vi "rszvl_core_global.vi"() -> ()   [LabVIEW 2014] (continued)
Callback"="", "Range Callback"="", "Check Callback"="", "Rngtable Callback"="", "Coerce Callback"="", "User Callback"="", "Supported Models"="", "Instrument Options"="", "Repeated Capabilities"="", "Restricted Repeated Capabilities"="", "Help"="This attribute sets the level when AM–modulated signals are used as trigger source.\n\nAvailable Repeated Capabilities:\nNone\n\nRemote-control command(s):\nTRIGger<1|2>[:SEQuence]:LEVel:AM:RELative", "Flags"={"OPC Wait"=FALSE, "Dont check status"=FALSE, "*WAI"=FALSE}, "Check Status Callback"=""}, {"Level"=2, "Descriptive Name"="Analog Demod Trigger FM Level", "Class Only"=FALSE, "Data Type"=1, "Access"=2, "Identifier"="RSZVL_ATTR_ADEM_TRIGGER_FM_LEVEL", "Range Table"="rszvl_rngAdemTrigFMLevel", "Command"="TRIG:LEV:FM", "Read Callback"="", "Write Callback"="", "Range Callback"="", "Check Callback"="", "Rngtable Callback"="", "Coerce Callback"="", "User Callback"="", "Supported Models"="", "Instrument Options"="", "Repeated Capabilities"="", "Restricted Repeated Capabilities"="", "Help"="This attribute sets the level when FM–modulated signals are used as trigger source.\n\nAvailable Repeated Capabilities:\nNone\n\nRemote-control command(s):\nTRIGger<1|2>[:SEQuence]:LEVel:FM", "Flags"={"OPC Wait"=FALSE, "Dont check status"=FALSE, "*WAI"=FALSE}, "Check Status Callback"=""}, {"Level"=2, "Descriptive Name"="Analog Demod Trigger PM Level", "Class Only"=FALSE, "Data Type"=1, "Access"=2, "Identifier"="RSZVL_ATTR_ADEM_TRIGGER_PM_LEVEL", "Range Table"="rszvl_rngAdemTrigPMLevel", "Command"="TRIG:LEV:PM", "Read Callback"="", "Write Callback"="", "Range Callback"="", "Check Callback"="", "Rngtable Callback"="", "Coerce Callback"="", "User Callback"="", "Supported Models"="", "Instrument Options"="", "Repeated Capabilities"="", "Restricted Repeated Capabilities"="", "Help"="This attribute sets the level when PM–modulated signals are used as trigger source.\n\nAvailable Repeated Capabilities:\nNone\n\nRemote-control command(s):\nTRIGger<1|2>[:SEQuence]:LEVel:PM", "Flags"={"OPC Wait"=FALSE, "Dont check status"=FALSE, "*WAI"=FALSE}, "Check Status Callback"=""}, {"Level"=2, "Descriptive Name"="Settings", "Class Only"=TRUE, "Data Type"=0, "Access"=0, "Identifier"="", "Range Table"="", "Command"="", "Read Callback"="", "Write Callback"="", "Range Callback"="", "Check Callback"="", "Rngtable Callback"="", "Coerce Callback"="", "User Callback"="", "Supported Models"="", "Instrument Options"="", "Repeated Capabilities"="", "Restricted Repeated Capabilities"="", "Help"="Attributes that configures the common settings of FM Demodulator.\n\n(1) FM Demod Display Pdiv:\nThis attribute defines the scaling of the Y axis in the current unit.\n\n(2) FM Demod State:\nThis attribute activates the FM demodulator of the instrument. The instrument will be set to timedomain\nmeasurement (span = 0) at the current center frequency. The detector will be set to\nSAMPle, the demodulator itself will be set up according to the parameters of command\n[SENSe:]ADEMod:SET.\n\n(3) FM Demod AF Coupling:\nThis attribute selects the coupling of the AF path.\n\n(4) FM Demod Meas Time:\nThis attribute sets the measuring time for the analog demodulation.\n\n(5) FM Demod Bandwidth:\nThis attribute defines the demodulation bandwidth for analog demodulation. Depending on the selected demodulation bandwidth, the instrument selects the required sampling rate.\nThe available values of the demodulation bandwidths are defined by the sampling rates.\n\n(6) FM Demod Record Length:\nThis attribute returns the currently set record length for the analog demodulation.\n\n(7) FM Demod Sampling Rate:\nThis attribute returns the currently set sampling rate for the analog demodulation.\n\n(8) FM Demod Zoom State:\nThis attribute switches on or off the zoom function for the trace data of the FM demodulator.\nDepending on the selected measuring time and demodulation bandwidth, more test points are recorded than can be displayed.\n\n(9) FM Demod Zoom Start:\nThis attribute selects the start time for the display of the single measured values of the FM\ndemodulator.\n\n(10) Analog Demod Phase Wrap:\nThis attribute activates the limitation to ±180°.\n\n(11) Analog Demod Unit Angle:\nThis attribute selects the unit for angles.\n\n(12) Analog Demod Zero Phase Ref Point:\nThis attribute activates the input of the reference point, where the phase is set to 0 rad.\n\n(13) Analog Demod THD Unit:\nThis attribute selects the unit for THD measurement results.", "Flags"={"OPC Wait"=FALSE, "Dont check status"=FALSE, "*WAI"=FALSE}, "Check Status Callback"=""}, {"Level"=3, "Descriptive Name"="FM Demod Display Pdiv", "Class Only"=FALSE, "Data Type"=1, "Access"=2, "Identifier"="RSZVL_ATTR_FMDEM_DISPLAY_PDIV", "Range Table"="", "Command"="DISP:WIND:TRAC:Y:PDIV", "Read Callback"="", "Write Callback"="", "Range Callback"="", "Check Callback"="", "Rngtable Callback"="", "Coerce Callback"="", "User Callback"="", "Supported Models"="", "Instrument Options"="", "Repeated Capabilities"="", "Restricted Repeated Capabilities"="", "Help"="This attribute defines the scaling of the Y axis in the current unit.\n\nAvailable Repeated Capabilities:\nNone\n\nRemote-control command(s):\nDISPlay[:WINDow<1|2>]:TRACE<1 to 3>:Y[:SCALe]:PDIVision", "Flags"={"OPC Wait"=FALSE, "Dont check status"=FALSE, "*WAI"=FALSE}, "Check Status Callback"=""}, {"Level"=3, "Descriptive Name"="FM Demod State", "Class Only"=FALSE, "Data Type"=3, "Access"=2, "Identifier"="RSZVL_ATTR_FMDEM_STATE", "Range Table"="", "Command"="ADEM", "Read Callback"="", "Write Callback"="", "Range Callback"="", "Check Callback"="", "Rngtable Callback"="", "Coerce Callback"="", "User Callback"="", "Supported Models"="", "Instrument Options"="", "Repeated Capabilities"="", "Restricted Repeated Capabilities"="", "Help"="This attribute activates the FM demodulator of the instrument. The instrument will be set to timedomain\nmeasurement (span = 0) at the current center frequency. The detector will be set to\nSAMPle, the demodulator itself will be set up according to the parameters of command\n[SENSe:]ADEMod:SET.\n\nAvailable Repeated Capabilities:\nNone\n\nRemote-control command(s):\n[SENSe:]ADEMod[:STATe] ON | OFF", "Flags"={"OPC Wait"=FALSE, "Dont check status"=FALSE, "*WAI"=FALSE}, "Check Status Callback"=""}, {"Level"=3, "Descriptive Name"="FM Demod AF Coupling", "Class Only"=FALSE, "Data Type"=0, "Access"=2, "Identifier"="RSZVL_ATTR_FMDEM_AF_COUP", "Range Table"="rszvl_rngCoupling", "Command"="ADEM:AF:COUP", "Read Callback"="", "Write Callback"="", "Range Callback"="", "Check Callback"="", "Rngtable Callback"="", "Coerce Callback"="", "User Callback"="", "Supported Models"="", "Instrument Options"="", "Repeated Capabilities"="", "Restricted Repeated Capabilities"="", "Help"="This attribute selects the coupling of the AF path.\n\nAvailable Repeated Capabilities:\nNone\n\nRemote-control command(s):\n[SENSe:]ADEMod:AF:COUPling AC | DC", "Flags"={"OPC Wait"=FALSE, "Dont check status"=FALSE, "*WAI"=FALSE}, "Check Status Callback"=""}, {"Level"=3, "Descriptive Name"="FM Demod Meas Time", "Class Only"=FALSE, "Data Type"=1, "Access"=2, "Identifier"="RSZVL_ATTR_FMDEM_MTIM", "Range Table"="", "Command"="ADEM:MTIM", "Read Callback"="", "Write Callback"="", "Range Callback"="", "Check Callback"="", "Rngtable Callback"="", "Coerce Callback"="", "User Callback"="", "Supported Models"="", "Instrument Options"="", "Repeated Capabilities"="", "Restricted Repeated Capabilities"="", "Help"="This attribute sets the measuring time for the analog demodulation.\n\nAvailable Repeated Capabilities:\nNone\n\nRemote-control command(s):\n[SENSe:]ADEMod:MTIMe", "Flags"={"OPC Wait"=FALSE, "Dont check status"=FALSE, "*WAI"=FALSE}, "Check Status Callback"=""}, {"Level"=3, "Descriptive Name"="FM Demod Bandwidth", "Class Only"=FALSE, "Data Type"=1, "Access"=2, "Identifier"="RSZVL_ATTR_FMDEM_BAND_DEM", "Range Table"="rszvl_rngFmBwid", "Command"="ADEM:BAND:DEM", "Read Callback"="", "Write Callback"="", "Range Callback"="", "Check Callback"="", "Rngtable Callback"="", "Coerce Callback"="", "User Callback"="", "Supported Models"="", "Instrument Options"="", "Repeated Capabilities"="", "Restricted Repeated Capabilities"="", "Help"="This attribute defines the demodulation bandwidth for analog demodulation. Depending on the selected demodulation bandwidth, the instrument selects the required sampling rate.\nThe available values of the demodulation bandwidths are defined by the sampling rates.\n\nAvailable Repeated Capabilities:\nNone\n\nRemote-control command(s):\n[SENSe:]ADEMod:BANDwidth | BWIDth:DEModulation", "Flags"={"OPC Wait"=FALSE, "Dont check status"=FALSE, "*WAI"=FALSE}, "Check Status Callback"=""}, {"Level"=3, "Descriptive Name"="FM Demod Record Length", "Class Only"=FALSE, "Data Type"=1, "Access"=0, "Identifier"="RSZVL_ATTR_FMDEM_RLEN", "Range Table"="", "Command"="ADEM:RLEN?", "Read Callback"="", "Write Callback"="", "Range Callback"="", "Check Callback"="", "Rngtable Callback"="", "Coerce Callback"="", "User Callback"="", "Supported Models"="", "Instrument Options"="", "Repeated Capabilities"="", "Restricted Repeated Capabilities"="", "Help"="This attribute returns the currently set record length for the analog demodulation.\n\nAvailable Repeated Capabilities:\nNone\n\nRemote-control command(s):\n[SENSe:]ADEMod:RLENgth?", "Flags"={"OPC Wait"=FALSE, "Dont check status"=FALSE, "*WAI"=FALSE}, "Check Status Callback"=""}, {"Level"=3, "Descriptive Name"="FM Demod Sampling Rate", "Class Only"=FALSE, "Data Type"=1, "Access"=0, "Identifier"="RSZVL_ATTR_FMDEM_SRATE", "Range Table"="", "Command"="ADEM:SRAT?", "Read Callback"="", "Write Callback"="", "Range Callback"="", "Check Callback"="", "Rngtable Callback"="", "Coerce Callback"="", "User Callback"="", "Supported Models"="", "Instrument Options"="", "Repeated Capabilities"="", "Restricted Repeated Capabilities"="", "Help"="This attribute returns the currently set sampling rate for the analog demodulation.\n\nAvailable Repeated Capabilities:\nNone\n\nRemote-control command(s):\n[SENSe:]ADEMod:SRATe?", "Flags"={"OPC Wait"=FALSE, "Dont check status"=FALSE, "*WAI"=FALSE}, "Check Status Callback"=""}, {"Level"=3, "Descriptive Name"="FM Demod Zoom State", "Class Only"=FALSE, "Data Type"=3, "Access"=2, "Identifier"="RSZVL_ATTR_FMDEM_ZOOM", "Range Table"="", "Command"="ADEM:ZOOM", "Read Callback"="", "Write Callback"="", "Range Callback"="", "Check Callback"="", "Rngtable Callback"="", "Coerce Callback"="", "User Callback"="", "Supported Models"="", "Instrument Options"="", "Repeated Capabilities"="", "Restricted Repeated Capabilities"="", "Help"="This attribute switches on or off the zoom function for the trace data of the FM demodulator.\nDepending on the selected measuring time and demodulation bandwidth, more test points are recorded than can be displayed.\n\nAvailable Repeated Capabilities:\nNone\n\nRemote-control command(s):\n[SENSe:]ADEMod:ZOOM[:STATe] ON | OFF", "Flags"={"OPC Wait"=FALSE, "Dont check status"=FALSE, "*WAI"=FALSE}, "Check Status Callback"=""}, {"Level"=3, "Descriptive Name"="FM Demod Zoom Start", "Class Only"=FALSE, "Data Type"=1, "Access"=2, "Identifier"="RSZVL_ATTR_FMDEM_ZOOM_START", "Range Table"="", "Command"="ADEM:ZOOM:STAR", "Read Callback"="", "Write Callback"="", "Range Callback"="", "Check Callback"="", "Rngtable Callback"="", "Coerce Callback"="", "User Callback"="", "Supported Models"="", "Instrument Options"="", "Repeated Capabilities"="", "Restricted Repeated Capabilities"="", "Help"="This attribute selects the start time for the display of the single measured values of the FM\ndemodulator.\n\nAvailable Repeated Capabilities:\nNone\n\nRemote-control command(s):\n[SENSe:]ADEMod:ZOOM:STARt", "Flags"={"OPC Wait"=FALSE, "Dont check status"=FALSE, "*WAI"=FALSE}, "Check Status Callback"=""}, {"Level"=3, "Descriptive Name"="Analog Demod Phase Wrap", "Class Only"=FALSE, "Data Type"=0, "Access"=2, "Identifier"="RSZVL_ATTR_ADEM_PHASE_WRAP", "Range Table"="rszvl_rngAdemPhaseWrap", "Command"="CALC:FORM", "Read Callback"="", "Write Callback"="", "Range Callback"="", "Check Callback"="", "Rngtable Callback"="", "Coerce Callback"="", "User Callback"="", "Supported Models"="", "Instrument Options"="", "Repeated Capabilities"="", "Restricted Repeated Capabilities"="", "Help"="This attribute activates the limitation to ±180°.\n\nAvailable Repeated Capabilities:\nNone\n\nRemote-control command(s):\nCALCulate<1|2>:FORMat", "Flags"={"OPC Wait"=FALSE, "Dont check status"=FALSE, "*WAI"=FALSE}, "Check Status Callback"=""}, {"Level"=3, "Descriptive Name"="Analog Demod Unit Angle", "Class Only"=FALSE, "Data Type"=0, "Access"=2, "Identifier"="RSZVL_ATTR_ADEM_UNIT_ANGLE", "Range Table"="rszvl_rngUnitAngle", "Command"="CALC:UNIT:ANGL", "Read Callback"="", "Write Callback"="", "Range Callback"="", "Check Callback"="", "Rngtable Callback"="", "Coerce Callback"="", "User Callback"="", "Supported Models"="", "Instrument Options"="", "Repeated Capabilities"="", "Restricted Repeated Capabilities"="", "Help"="This attribute selects the unit for angles.\n\nAvailable Repeated Capabilities:\nNone\n\nRemote-control command(s):\nCALCulate<1|2>:UNIT:ANGLe", "Flags"={"OPC Wait"=FALSE, "Dont check status"=FALSE, "*WAI"=FALSE}, "Check Status Callback"=""}, {"Level"=3, "Descriptive Name"="Analog Demod Zero Phase Ref Point", "Class Only"=FALSE, "Data Type"=1, "Access"=2, "Identifier"="RSZVL_ATTR_ADEM_PM_RPO_X", "Range Table"="", "Command"="ADEM:PM:RPO:X", "Read Callback"="", "Write Callback"="", "Range Callback"="", "Check Callback"="", "Rngtable Callback"="", "Coerce Callback"="", "User Callback"="", "Supported Models"="", "Instrument Options"="", "Repeated Capabilities"="", "Restricted Repeated Capabilities"="", "Help"="This attribute activates the input of the reference point, where the phase is set to 0 rad.\n\nAvailable Repeated Capabilities:\nNone\n\nRemote-control command(s):\n[SENSe1:]ADEMod:PM:RPO:X", "Flags"={"OPC Wait"=FALSE, "Dont check status"=FALSE, "*WAI"=FALSE}, "Check Status Callback"=""}, {"Level"=2, "Descriptive Name"="AF Frequency Settings", "Class Only"=TRUE, "Data Type"=0, "Access"=0, "Identifier"="", "Range Table"="", "Command"="", "Read Callback"="", "Write Callback"="", "Range Callback"="", "Check Callback"="", "Rngtable Callback"="", "Coerce Callback"="", "User Callback"="", "Supported Models"="", "Instrument Options"="", "Repeated Capabilities"="", "Restricted Repeated Capabilities"="", "Help"="Attributes that configures the AF Frequency settings.\n\n(1) FM Demod AF Center Frequency:\nThis attribute sets the center frequency for result display AF spectrum.\n\n(2) FM Demod AF Span:\nThis attribute sets the span for result display AF spectrum.\nThe span is limited to half the measurement bandwidth of analog demodulation.\n\n(3) FM Demod AF Start Frequency:\nThis attribute sets the start frequency for result display AF spectrum.\n\n(4) FM Demod AF Stop Frequency:\nThis attribute sets the stop frequency for result display AF spectrum.\nThe stop frequency is limited to half the measurement bandwidth of analog demodulation.\n\n(5) FM Demod AF Full Span:\nThis attribute sets the maximum span for the display of the AF spectrum.", "Flags"={"OPC Wait"=FALSE, "Dont check status"=FALSE, "*WAI"=FALSE}, "Check Status Callback"=""}, {"Level"=3, "Descriptive Name"="FM Demod AF Center Frequency", "Class Only"=FALSE, "Data Type"=1, "Access"=2, "Identifier"="RSZVL_ATTR_FMDEM_AF_CENTER", "Range Table"="", "Command"="ADEM:AF:CENT", "Read Callback"="", "Write Callback"="", "Range Callback"="", "Check Callback"="", "Rngtable Callback"="", "Coerce Callback"="", "User Callback"="", "Supported Models"="", "Instrument Options"="", "Repeated Capabilities"="", "Restricted Repeated Capabilities"="", "Help"="This attribute sets the center frequency for result display AF spectrum.\n\nAvailable Repeated Capabilities:\nNone\n\nRemote-control command(s):\n[SENSe:]ADEMod:AF:CENTer", "Flags"={"OPC Wait"=FALSE, "Dont check status"=FALSE, "*WAI"=FALSE}, "Check Status Callback"=""}, {"Level"=3, "Descriptive Name"="FM Demod AF Span", "Class Only"=FALSE, "Data Type"=1, "Access"=2, "Identifier"="RSZVL_ATTR_FMDEM_AF_SPAN", "Range Table"="", "Command"="ADEM:AF:SPAN", "Read Callback"="", "Write Callback"="", "Range Callback"="", "Check Callback"="", "Rngtable Callback"="", "Coerce Callback"="", "User Callback"="", "Supported Models"="", "Instrument Options"="", "Repeated Capabilities"="", "Restricted Repeated Capabilities"="", "Help"="This attribute sets the span for result display AF spectrum.\nThe span is limited to half the measurement bandwidth of analog demodulation.\n\nAvailable Repeated Capabilities:\nNone\n\nRemote-control command(s):\n[SENSe:]ADEMod:AF:SPAN", "Flags"={"OPC Wait"=FALSE, "Dont check status"=FALSE, "*WAI"=FALSE}, "Check Status Callback"=""}, {"Level"=3, "Descriptive Name"="FM Demod AF Start Frequency", "Class Only"=FALSE, "Data Type"=1, "Access"=2, "Identifier"="RSZVL_ATTR_FMDEM_AF_START", "Range Table"="", "Command"="ADEM:AF:STAR", "Read Callback"="", "Write Callback"="", "Range Callback"="", "Check Callback"="", "Rngtable Callback"="", "Coerce Callback"="", "User Callback"="", "Supported Models"="", "Instrument Options"="", "Repeated Capabilities"="", "Restricted Repeated Capabilities"="", "Help"="This attribute sets the start frequency for result display AF spectrum.\n\nAvailable Repeated Capabilities:\nNone\n\nRemote-control command(s):\n[SENSe:]ADEMod:AF:STARt", "Flags"={"OPC Wait"=FALSE, "Dont check status"=FALSE, "*WAI"=FALSE}, "Check Status Callback"=""}, {"Level"=3, "Descriptive Name"="FM Demod AF Stop Frequency", "Class Only"=FALSE, "Data Type"=1, "Access"=2, "Identifier"="RSZVL_ATTR_FMDEM_AF_STOP", "Range Table"="", "Command"="ADEM:AF:STOP", "Read Callback"="", "Write Callback"="", "Range Callback"="", "Check Callback"="", "Rngtable Callback"="", "Coerce Callback"="", "User Callback"="", "Supported Models"="", "Instrument Options"="", "Repeated Capabilities"="", "Restricted Repeated Capabilities"="", "Help"="This attribute sets the stop frequency for result display AF spectrum.\nThe stop frequency is limited to half the measurement bandwidth of analog demodulation.\n\nAvailable Repeated Capabilities:\nNone\n\nRemote-control command(s):\n[SENSe:]ADEMod:AF:STOP", "Flags"={"OPC Wait"=FALSE, "Dont check status"=FALSE, "*WAI"=FALSE}, "Check Status Callback"=""}, {"Level"=3, "Descriptive Name"="FM Demod AF Full Span", "Class Only"=FALSE, "Data Type"=4, "Access"=1, "Identifier"="RSZVL_ATTR_FMDEM_AF_FULL_SPAN", "Range Table"="", "Command"="ADEM:AF:SPAN:FULL", "Read Callback"="", "Write Callback"="", "Range Callback"="", "Check Callback"="", "Rngtable Callback"="", "Coerce Callback"="", "User Callback"="", "Supported Models"="", "Instrument Options"="", "Repeated Capabilities"="", "Restricted Repeated Capabilities"="", "Help"="This attribute sets the maximum span for the display of the AF spectrum.\n\nAvailable Repeated Capabilities:\nNone\n\nRemote-control command(s):\n[SENSe:]ADEMod:AF:SPAN:FULL", "Flags"={"OPC Wait"=FALSE, "Dont check status"=FALSE, "*WAI"=FALSE}, "Check Status Callback"=""}, {"Level"=2, "Descriptive Name"="RF Spectrum Settings", "Class Only"=TRUE, "Data Type"=0, "Access"=0, "Identifier"="", "Range Table"="", "Command"="", "Read Callback"="", "Write Callback"="", "Range Callback"="", "Check Callback"="", "Rngtable Callback"="", "Coerce Callback"="", "User Callback"="", "Supported Models"="", "Instrument Options"="", "Repeated Capabilities"="", "Restricted Repeated Capabilities"="", "Help"="Attributes that configures the RF Spectrum settings.\n\n(1) FM Demod RF Spectrum Resolution Bandwidth:\nThis attribute sets the resolution bandwidth for display of the RF spectrum from the data of analog\ndemodulation.\nThe required record length is calculated from the sampling rate directly set via\nADEM:SPEC:SPAN:MAX or ADEM:BAND. If the available record length is not sufficient for the\ngiven bandwidth, it is set to maximum and the resolution bandwidth is increased accordingly.\n\n(2) FM Demod RF Spectrum Span:\nThis attribute sets the maximum frequency range for result display of RF spectrum resulting from\nthe FM demodulation data. The maximum span corresponds to the measurement bandwidth of\nanalog demodulation (SENS:ADEM:BAND).\n\n(3) FM Demod RF Spectrum Zoom:\nThis attribute sets the frequency range for result display of RF spectrum determined from FM demodulation data. The frequency range for result display is limited to the maximum span or to the measurement  bandwidth of analog demodulation.", "Flags"={"OPC Wait"=FALSE, "Dont check status"=FALSE, "*WAI"=FALSE}, "Check Status Callback"=""}, {"Level"=3, "Descriptive Name"="FM Demod RF Spectrum Resolution Bandwidth", "Class Only"=FALSE, "Data Type"=1, "Access"=2, "Identifier"="RSZVL_ATTR_FMDEM_BAND_RES", "Range Table"="rszvl_rngAdemBandRes", "Command"="ADEM:SPEC:BAND", "Read Callback"="", "Write Callback"="", "Range Callback"="", "Check Callback"="", "Rngtable Callback"="", "Coerce Callback"="", "User Callback"="", "Supported Models"="", "Instrument Options"="", "Repeated Capabilities"="", "Restricted Repeated Capabilities"="", "Help"="This attribute sets the resolution bandwidth for display of the RF spectrum from the data of analog\ndemodulation.\nThe required record length is calculated from the sampling rate directly set via\nADEM:SPEC:SPAN:MAX or ADEM:BAND. If the available record length is not sufficient for the\ngiven bandwidth, it is set to maximum and the resolution bandwidth is increased accordingly.\n\nAvailable Repeated Capabilities:\nNone\n\nRemote-control command(s):\n[SENSe:]ADEMod:SPECtrum:BANDwidth|BWIDth[:RESolution]", "Flags"={"OPC Wait"=FALSE, "Dont check status"=FALSE, "*WAI"=FALSE}, "Check Status Callback"=""}, {"Level"=3, "Descriptive Name"="FM Demod RF Spectrum Span", "Class Only"=FALSE, "Data Type"=1, "Access"=2, "Identifier"="RSZVL_ATTR_FMDEM_SPEC_SPAN", "Range Table"="", "Command"="ADEM:SPEC:SPAN", "Read Callback"="", "Write Callback"="", "Range Callback"="", "Check Callback"="", "Rngtable Callback"="", "Coerce Callback"="", "User Callback"="", "Supported Models"="", "Instrument Options"="", "Repeated Capabilities"="", "Restricted Repeated Capabilities"="", "Help"="This attribute sets the maximum frequency range for result display of RF spectrum resulting from\nthe FM demodulation data. The maximum span corresponds to the measurement bandwidth of\nanalog demodulation (SENS:ADEM:BAND).\n\nAvailable Repeated Capabilities:\nNone\n\nRemote-control command(s):\n[SENSe:]ADEMod:SPECtrum:SPAN[:MAXimum]", "Flags"={"OPC Wait"=FALSE, "Dont check status"=FALSE, "*WAI"=FALSE}, "Check Status Callback"=""}, {"Level"=3, "Descriptive Name"="FM Demod RF Spectrum Zoom", "Class Only"=FALSE, "Data Type"=1, "Access"=2, "Identifier"="RSZVL_ATTR_FMDEM_SPEC_ZOOM", "Range Table"="", "Command"="ADEM:SPEC:SPAN:ZOOM", "Read Callback"="", "Write Callback"="", "Range Callback"="", "Check Callback"="", "Rngtable Callback"="", "Coerce Callback"="", "User Callback"="", "Supported Models"="", "Instrument Options"="", "Repeated Capabilities"="", "Restricted Repeated Capabilities"="", "Help"="This attribute sets the frequency range for result display of RF spectrum determined from FM demodulation data. The frequency range for result display is limited to the maximum span or to the measurement  bandwidth of analog demodulation.\n\nAvailable Repeated Capabilities:\nNone\n\nRemote-control command(s):\n[SENSe:]ADEMod:SPECtrum:SPAN:ZOOM", "Flags"={"OPC Wait"=FALSE, "Dont check status"=FALSE, "*WAI"=FALSE}, "Check Status Callback"=""}, {"Level"=2, "Descriptive Name"="AF Filter Settings", "Class Only"=TRUE, "Data Type"=0, "Access"=0, "Identifier"="", "Range Table"="", "Command"="", "Read Callback"="", "Write Callback"="", "Range Callback"="", "Check Callback"="", "Rngtable Callback"="", "Coerce Callback"="", "User Callback"="", "Supported Models"="", "Instrument Options"="", "Repeated Capabilities"="", "Restricted Repeated Capabilities"="", "Help"="Attributes that configures the AF Filter settings.\n\n(1) FM Demod High Pass AF Filter State:\nThis attribute switches on a high pass filter with the given limit to separate the DC component.\n\n(2) FM Demod High Pass AF Filter Frequency:\nThis attribute sets the limit of high pass filter to separate the DC component. The filters are indicated by the 3 dB cutoff frequency. The filters are designed as 2nd-order Butterworth filter (12 dB/octave).\n\n(3) FM Demod Low Pass AF Filter State:\nThis attribute switches on/off a low pass filter.\n\n(4) FM Demod Deemphasis State:\nThis attribute switches on/off the de-emphasis.\n\n(5) FM Demod Low Pass AF Filter Frequency:\nThis attribute sets the limit of low pass filter. The filter are indicated by the 3 dB cutoff frequency. The 3 kHz and 15 kHz filters are designed as 5th-order Butterworth filter (30 dB/octave). The\n150 kHz filter is designed as 8th-order Butterworth filter (48 dB/octave).\n\n(6) FM Demod Deemphasis Time Constant:\nThis attribute sets the de-emphasisi time constant.\n\n(7) Analog Demod Low Pass Filter Frequency Relative:\nThis attribute selects the relative low pass filter type.\n\n(8) Analog Demod Filter CCITT Weighting:\nThis attribute activates/deactivate CCITT filter weightening. \nCCITT 25 kHz <= demodulation bandwidth <= 3 MHz\n\n(9) Analog Demod Filter CCIR Weighting:\nThis attribute activates/deactivate CCIR filter weightening. \nCCIR 50 kHz <= demodulation bandwidth <= 1.6 MHz", "Flags"={"OPC Wait"=FALSE, "Dont check status"=FALSE, "*WAI"=FALSE}, "Check Status Callback"=""}, {"Level"=3, "Descriptive Name"="FM Demod High Pass AF Filter State", "Class Only"=FALSE, "Data Type"=3, "Access"=2, "Identifier"="RSZVL_ATTR_FMDEM_FILT_HPAS_STAT", "Range Table"="", "Command"="FILT:HPAS", "Read Callback"="", "Write Callback"="", "Range Callback"="", "Check Callback"="", "Rngtable Callback"="", "Coerce Callback"="", "User Callback"="", "Supported Models"="", "Instrument Options"="", "Repeated Capabilities"="", "Restricted Repeated Capabilities"="", "Help"="This attribute switches on a high pass filter with the given limit to separate the DC component.\n\nAvailable Repeated Capabilities:\nNone\n\nRemote-control command(s):\n[SENSe:]FILTer:HPASs[:STATe] ON | OFF", "Flags"={"OPC Wait"=FALSE, "Dont check status"=FALSE, "*WAI"=FALSE}, "Check Status Callback"=""}, {"Level"=3, "Descriptive Name"="FM Demod High Pass AF Filter Frequency", "Class Only"=FALSE, "Data Type"=1, "Access"=2, "Identifier"="RSZVL_ATTR_FMDEM_FILT_HPAS_FREQ", "Range Table"="rszvl_rngHpasFilterFreq", "Command"="FILT:HPAS:FREQ", "Read Callback"="", "Write Callback"="", "Range Callback"="", "Check Callback"="", "Rngtable Callback"="", "Coerce Callback"="", "User Callback"="", "Supported Models"="", "Instrument Options"="", "Repeated Capabilities"="", "Restricted Repeated Capabilities"="", "Help"="This attribute sets the limit of high pass filter to separate the DC component. The filters are indicated by the 3 dB cutoff frequency. The filters are designed as 2nd-order Butterworth filter (12 dB/octave).\n\nAvailable Repeated Capabilities:\nNone\n\nRemote-control command(s):\n[SENSe:]FILTer:HPASs:FREQuency 50 Hz | 300 Hz", "Flags"={"OPC Wait"=FALSE, "Dont check status"=FALSE, "*WAI"=FALSE}, "Check Status Callback"=""}, {"Level"=3, "Descriptive Name"="FM Demod Low Pass AF Filter State", "Class Only"=FALSE, "Data Type"=3, "Access"=2, "Identifier"="RSZVL_ATTR_FMDEM_FILT_LPAS_STAT", "Range Table"="", "Command"="FILT:LPAS", "Read Callback"="", "Write Callback"="", "Range Callback"="", "Check Callback"="", "Rngtable Callback"="", "Coerce Callback"="", "User Callback"="", "Supported Models"="", "Instrument Options"="", "Repeated Capabilities"="", "Restricted Repeated Capabilities"="", "Help"="This attribute switches on/off a low pass filter.\n\nAvailable Repeated Capabilities:\nNone\n\nRemote-control command(s):\n[SENSe:]FILTer:LPASs[:STATe] ON | OFF", "Flags"={"OPC Wait"=FALSE, "Dont check status"=FALSE, "*WAI"=FALSE}, "Check Status Callback"=""}, {"Level"=3, "Descriptive Name"="FM Demod Deemphasis State", "Class Only"=FALSE, "Data Type"=3, "Access"=2, "Identifier"="RSZVL_ATTR_FMDEM_FILT_DEMP_STAT", "Range Table"="", "Command"="FILT:DEMP", "Read Callback"="", "Write Callback"="", "Range Callback"="", "Check Callback"="", "Rngtable Callback"="", "Coerce Callback"="", "User Callback"="", "Supported Models"="", "Instrument Options"="", "Repeated Capabilities"="", "Restricted Repeated Capabilities"="", "Help"="This attribute switches on/off the de-emphasis.\n\nAvailable Repeated Capabilities:\nNone\n\nRemote-control command(s):\n[SENSe:]FILTer:DEMPhasis[:STATe] ON | OFF", "Flags"={"OPC Wait"=FALSE, "Dont check status"=FALSE, "*WAI"=FALSE}, "Check Status Callback"=""}, {"Level"=3, "Descriptive Name"="FM Demod Low Pass AF Filter Frequency", "Class Only"=FALSE, "Data Type"=1, "Access"=2, "Identifier"="RSZVL_ATTR_FMDEM_FILT_LPAS_FREQ", "Range Table"="rszvl_rngLpasFiltFreq", "Command"="FILT:LPAS:FREQ", "Read Callback"="", "Write Callback"="", "Range Callback"="", "Check Callback"="", "Rngtable Callback"="", "Coerce Callback"="", "User Callback"="", "Supported Models"="", "Instrument Options"="", "Repeated Capabilities"="", "Restricted Repeated Capabilities"="", "Help"="This attribute sets the limit of low pass filter. The filter are indicated by the 3 dB cutoff frequency. The 3 kHz and 15 kHz filters are designed as 5th-order Butterworth filter (30 dB/octave). The\n150 kHz filter is designed as 8th-order Butterworth filter (48 dB/octave).\n\nAvailable Repeated Capabilities:\nNone\n\nRemote-control command(s):\n[SENSe:]FILTer:LPASs:FREQuency 3 kHz | 15 kHz | 150 kHz", "Flags"={"OPC Wait"=FALSE, "Dont check status"=FALSE, "*WAI"=FALSE}, "Check Status Callback"=""}, {"Level"=3, "Descriptive Name"="FM Demod Deemphasis Time Constant", "Class Only"=FALSE, "Data Type"=1, "Access"=2, "Identifier"="RSZVL_ATTR_FMDEM_FILT_DEMP_TCON", "Range Table"="rszvl_rngFiltDempTimeConst", "Command"="FILT:DEMP:TCON", "Read Callback"="", "Write Callback"="", "Range Callback"="", "Check Callback"="", "Rngtable Callback"="", "Coerce Callback"="", "User Callback"="", "Supported Models"="", "Instrument Options"="", "Repeated Capabilities"="", "Restricted Repeated Capabilities"="", "Help"="This attribute sets the de-emphasisi time constant.\n\nAvailable Repeated Capabilities:\nNone\n\nRemote-control command(s):\n[SENSe:]FILTer:DEMPhasis:TCONstant 25 us | 50 us | 75 us | 750 us", "Flags"={"OPC Wait"=FALSE, "Dont check status"=FALSE, "*WAI"=FALSE}, "Check Status Callback"=""}, {"Level"=3, "Descriptive Name"="Analog Demod Low Pass Filter Frequency Relative", "Class Only"=FALSE, "Data Type"=0, "Access"=2, "Identifier"="RSZVL_ATTR_ADEM_FILT_LPAS_FREQ_REL", "Range Table"="rszvl_rngFiltDempPctConst", "Command"="SENS:FILT:LPAS:FREQ:REL", "Read Callback"="", "Write Callback"="", "Range Callback"="", "Check Callback"="", "Rngtable Callback"="", "Coerce Callback"="", "User Callback"="", "Supported Models"="", "Instrument Options"="", "Repeated Capabilities"="", "Restricted Repeated Capabilities"="", "Help"="This attribute selects the relative low pass filter type.\n\nAvailable Repeated Capabilities:\nNone\n\nRemote-control command(s):\n[SENSe<1|2>:]FILTer:LPASs:FREQuency:RELative", "Flags"={"OPC Wait"=FALSE, "Dont check status"=FALSE, "*WAI"=FALSE}, "Check Status Callback"=""}, {"Level"=2, "Descriptive Name"="Results", "Class Only"=TRUE, "Data Type"=0, "Access"=0, "Identifier"="", "Range Table"="", "Command"="", "Read Callback"="", "Write Callback"="", "Range Callback"="", "Check Callback"="", "Rngtable Callback"="", "Coerce Callback"="", "User Callback"="", "Supported Models"="", "Instrument Options"="", "Repeated Capabilities"="", "Restricted Repeated Capabilities"="", "Help"="Attributes that return the measurement results.\n\n(1) FM Demod Audio Frequency Result:\nThis attribute queries the audio frequency with analog demodulation.\n\n(2) FM Demod Frequency Error Result:\nThis attribute queries the frequency error with FM demodulation.\n\n(3) FM Demod SINAD Measurement Result:\nThis attribute queries the result of the SINAD measurement.\n\n(4) FM Demod THD Measurement Result:\nThis attribute queries the result of the THD measurement.\n\n(5) FM Demod Carrier Power Result:\nThis attribute queries the carrier power.\n\nWith result display FM and SPECTRUM, the carrier power is determined from the current trace data\n(CLR/WRITE trace).\nWith result display RF power, the carrier power is determined from trace 1 to 3 indicated in the\nnumeric suffix.\n\n(6) Analog Demod Summary Result Value:\nThis attribute queries the result od AM, FM or PM modulation measurement.\n\n(7) Analog Demod FM Offset:\nThis attribute calculates the FM offset of the current measured data set.", "Flags"={"OPC Wait"=FALSE, "Dont check status"=FALSE, "*WAI"=FALSE}, "Check Status Callback"=""}, {"Level"=3, "Descriptive Name"="FM Demod Audio Frequency Result", "Class Only"=FALSE, "Data Type"=1, "Access"=0, "Identifier"="RSZVL_ATTR_FMDEM_AFR_RES", "Range Table"="", "Command"="CALC:MARK:FUNC:ADEM:AFR:RES{Trace}?", "Read Callback"="", "Write Callback"="", "Range Callback"="", "Check Callback"="", "Rngtable Callback"="", "Coerce Callback"="", "User Callback"="", "Supported Models"="", "Instrument Options"="", "Repeated Capabilities"="", "Restricted Repeated Capabilities"="", "Help"="This attribute queries the audio frequency with analog demodulation.\n\nAvailable Repeated Capabilities:\nTrace: TR1,TR2,TR3,TR4,TR5,TR6,TR7,TR8,TR9,TR10,TR11,TR12,TR13,TR14,TR15,TR16,TR17,TR18,TR19,TR20\r\n\nRemote-control command(s):\nCALCulate<1|2>:MARKer:FUNCtion:ADEMod:AFRequency[:RESult<1...4>]?", "Flags"={"OPC Wait"=FALSE, "Dont check status"=FALSE, "*WAI"=FALSE}, "Check Status Callback"=""}, {"Level"=3, "Descriptive Name"="FM Demod Frequency Error Result", "Class Only"=FALSE, "Data Type"=1, "Access"=0, "Identifier"="RSZVL_ATTR_FMDEM_FERR_RES", "Range Table"="", "Command"="CALC:MARK:FUNC:ADEM:FERR:RES{Trace}?", "Read Callback"="", "Write Callback"="", "Range Callback"="", "Check Callback"="", "Rngtable Callback"="", "Coerce Callback"="", "User Callback"="", "Supported Models"="", "Instrument Options"="", "Repeated Capabilities"="", "Restricted Repeated Capabilities"="", "Help"="This attribute queries the frequency error with FM demodulation.\n\nAvailable Repeated Capabilities:\nTrace: TR1,TR2,TR3,TR4,TR5,TR6,TR7,TR8,TR9,TR10,TR11,TR12,TR13,TR14,TR15,TR16,TR17,TR18,TR19,TR20\r\n\nRemote-control command(s):\nCALCulate<1|2>:MARKer:FUNCtion:ADEMod:FERRor[:RESult<1...4>]?", "Flags"={"OPC Wait"=FALSE, "Dont check status"=FALSE, "*WAI"=FALSE}, "Check Status Callback"=""}, {"Level"=3, "Descriptive Name"="FM Demod SINAD Measurement Result", "Class Only"=FALSE, "Data Type"=1, "Access"=0, "Identifier"="RSZVL_ATTR_FMDEM_SIN_RES", "Range Table"="", "Command"="CALC:MARK:FUNC:ADEM:SIN:RES{Trace}?", "Read Callback"="", "Write Callback"="", "Range Callback"="", "Check Callback"="", "Rngtable Callback"="", "Coerce Callback"="", "User Callback"="", "Supported Models"="", "Instrument Options"="", "Repeated Capabilities"="", "Restricted Repeated Capabilities"="", "Help"="This attribute queries the result of the SINAD measurement.\n\nAvailable Repeated Capabilities:\nTrace: TR1,TR2,TR3,TR4,TR5,TR6,TR7,TR8,TR9,TR10,TR11,TR12,TR13,TR14,TR15,TR16,TR17,TR18,TR19,TR20\r\n\nRemote-control command(s):\nCALCulate<1|2>:MARKer:FUNCtion:ADEMod:SINad:RESult<1...4>?", "Flags"={"OPC Wait"=FALSE, "Dont check status"=FALSE, "*WAI"=FALSE}, "Check Status Callback"=""}, {"Level"=3, "Descriptive Name"="FM Demod THD Measurement Result", "Class Only"=FALSE, "Data Type"=1, "Access"=0, "Identifier"="RSZVL_ATTR_FMDEM_THD_RES", "Range Table"="", "Command"="CALC:MARK:FUNC:ADEM:THD:RES{Trace}?", "Read Callback"="", "Write Callback"="", "Range Callback"="", "Check Callback"="", "Rngtable Callback"="", "Coerce Callback"="", "User Callback"="", "Supported Models"="", "Instrument Options"="", "Repeated Capabilities"="", "Restricted Repeated Capabilities"="", "Help"="This attribute queries the result of the THD measurement.\n\nAvailable Repeated Capabilities:\nTrace: TR1,TR2,TR3,TR4,TR5,TR6,TR7,TR8,TR9,TR10,TR11,TR12,TR13,TR14,TR15,TR16,TR17,TR18,TR19,TR20\r\n\nRemote-control command(s):\nCALCulate<1|2>:MARKer:FUNCtion:ADEMod:THD:RESult<1...4>?", "Flags"={"OPC Wait"=FALSE, "Dont check status"=FALSE, "*WAI"=FALSE}, "Check Status Callback"=""}, {"Level"=3, "Descriptive Name"="FM Demod Carrier Power Result", "Class Only"=FALSE, "Data Type"=1, "Access"=0, "Identifier"="RSZVL_ATTR_FMDEM_CARR_RES", "Range Table"="", "Command"="CALC:MARK:FUNC:ADEM:CARR:RES{Trace}?", "Read Callback"="", "Write Callback"="", "Range Callback"="", "Check Callback"="", "Rngtable Callback"="", "Coerce Callback"="", "User Callback"="", "Supported Models"="", "Instrument Options"="", "Repeated Capabilities"="", "Restricted Repeated Capabilities"="", "Help"="This attribute queries the carrier power.\n\nWith result display FM and SPECTRUM, the carrier power is determined from the current trace data\n(CLR/WRITE trace).\nWith result display RF power, the carrier power is determined from trace 1 to 3 indicated in the\nnumeric suffix.\n\nAvailable Repeated Capabilities:\nTrace: TR1,TR2,TR3,TR4,TR5,TR6,TR7,TR8,TR9,TR10,TR11,TR12,TR13,TR14,TR15,TR16,TR17,TR18,TR19,TR20\r\n\nRemote-control command(s):\nCALCulate<1|2>:MARKer:FUNCtion:ADEMod:CARRier[:RESult<1...4>]?", "Flags"={"OPC Wait"=FALSE, "Dont check status"=FALSE, "*WAI"=FALSE}, "Check Status Callback"=""}, {"Level"=3, "Descriptive Name"="Analog Demod Summary Result Value", "Class Only"=FALSE, "Data Type"=1, "Access"=0, "Identifier"="RSZVL_ATTR_ADEM_SUMM_RES", "Range Table"="", "Command"="CALC:MARK:FUNC:ADEM:{AnalogModulation}:RES{Trace}? {ResultDetector}", "Read Callback"="", "Write Callback"="", "Range Callback"="", "Check Callback"="", "Rngtable Callback"="", "Coerce Callback"="", "User Callback"="", "Supported Models"="", "Instrument Options"="", "Repeated Capabilities"="", "Restricted Repeated Capabilities"="", "Help"="This attribute queries the result od AM, FM or PM modulation measurement.\n\nAvailable Repeated Capabilities:\nAnalogModulation: AnalogAM,AnalogFM,AnalogPM\r\nTrace: TR1,TR2,TR3,TR4,TR5,TR6,TR7,TR8,TR9,TR10,TR11,TR12,TR13,TR14,TR15,TR16,TR17,TR18,TR19,TR20\r\nResultDetector: ResDetPosPeak,ResDetNegPeak,ResDetAverPeak,ResDetRMS\r\n\nRemote-control command(s):\nCALCulate<1|2>:MARKer:FUNCtion:ADEMod:AM|FM|PM[:RESult<1...4>?] PPEak | MPEak | MIDDle | RMS", "Flags"={"OPC Wait"=FALSE, "Dont check status"=FALSE, "*WAI"=FALSE}, "Check Status Callback"=""}, {"Level"=3, "Descriptive Name"="Analog Demod FM Offset", "Class Only"=FALSE, "Data Type"=1, "Access"=0, "Identifier"="RSZVL_ATTR_ADEM_FM_OFFSET", "Range Table"="", "Command"="ADEM:FM:OFFS? {FMOffsetResult}", "Read Callback"="", "Write Callback"="", "Range Callback"="", "Check Callback"="", "Rngtable Callback"="", "Coerce Callback"="", "User Callback"="", "Supported Models"="", "Instrument Options"="", "Repeated Capabilities"="", "Restricted Repeated Capabilities"="", "Help"="This attribute calculates the FM offset of the current measured data set.\n\nAvailable Repeated Capabilities:\nFMOffsetResult: FMOffImm,FMOffAver\r\n\nRemote-control command(s):\n[SENSe:]ADEMod:FM:OFFSet? IMMediate | AVERage", "Flags"={"OPC Wait"=FALSE, "Dont check status"=FALSE, "*WAI"=FALSE}, "Check Status Callback"=""}, {"Level"=1, "Descriptive Name"="K8 - Bluetooth Analyzer", "Class Only"=TRUE, "Data Type"=0, "Access"=0, "Identifier"="", "Range Table"="", "Command"="", "Read Callback"="", "Write Callback"="", "Range Callback"="", "Check Callback"="", "Rngtable Callback"="", "Coerce Callback"="", "User Callback"="", "Supported Models"="", "Instrument Options"="", "Repeated Capabilities"="", "Restricted Repeated Capabilities"="", "Help"="This class defines attributes of Bluetooth Measurements\n\n(1) Settings (Class):\nAttributes that configure 
